vi "纳清pH电极校准.vi"() -> ()   [LabVIEW 2016, in "斯坦道多参数.lvlib"]
uses:
  <vilib>/Utility/miscctls.llb/LVPointTypeDef.ctl
  <vilib>/Utility/miscctls.llb/LVPositionTypeDef.ctl
  <vilib>/Analysis/NI_AALBase.lvlib
panel:
  out "当前探头类别":string
  out "报警信息":string
  out "温度校准参数":sgl format="%#.2f"
  out "通讯状态":string
  out "第二点校准值":dbl
  out "第一点校准值":dbl
  in  "校准停止":bool
  in  "校准启动":bool
  in  "校准模式":enum16{"两点校准", "单点校准"}(ring)
  out "最小值":sgl format="%#.2f"
  out "最大值":sgl format="%#.2f"
  out "波形图表":sgl(graph) caption="历史曲线"
  out "mean":dbl caption="均值" format="%#.2f"
  out "standard deviation":dbl caption="标准差" format="%#.2f"
  out "变异系数":dbl format="%#.6f"
  out "测量值":sgl format="%#.2f"
  out "提示":string
  out "标液2":sgl
  out "标液1":sgl
  out "原始光强数值":sgl caption="信号值" format="%#.6f"
  out "温度":dbl format="%#.2f"
  # "pH电极设定"
  # "℃"
  # "mV"
  # "℃"
  # "请选择校准模式:"
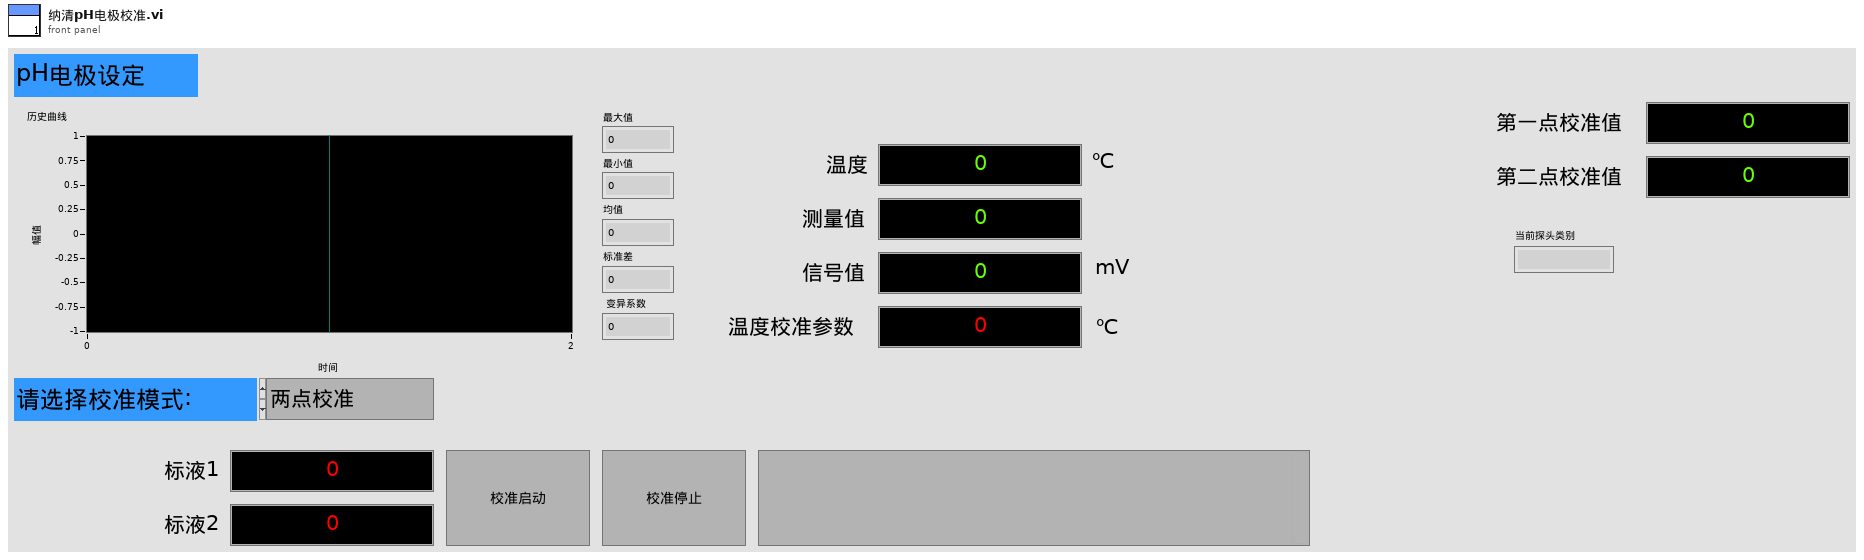
[diagram p1: front panel]
types:
  T1 = typedef "LVPointTypeDef.ctl" = cluster{"Horizontal":i16, "Vertical":i16}
  T2 = typedef "斯坦道多参数.lvlib/校准步骤.ctl" = enum16{"待机", "放置第一点标液", "第一点校准启动", "第一点校准写入", "第一点校准失败", "放置第二点标液", "第二点校准启动", "第二点校准写入", "第二点校准失败", "放置第三点标液", "第三点校准启动", "第三点校准写入", "第三点校准失败", "校准结果写入", "校准结束"}
  T3 = cluster{"报警码":u16, "pH数值":sgl, "0X0003_NC":sgl, "温度数据":sgl, "pH原始信号 mv":sgl, "0X0009_NC":string, "产品名称":string, "序列号":string, "硬件版本":string, "软件版本":string, "通讯地址":u16, "波特率":u16, "设备类型":u16, "0X0026_NC":string, "第一点原始数据":sgl, "第一点校准数据":sgl, "第二点原始数据":sgl, "第二点校准数据":sgl, "探头校准命令":u16, "温度校准参数":sgl, "温度校准命令":u16}
  T4 = typedef "LVPositionTypeDef.ctl" = cluster{"Left":i32, "Top":i32}
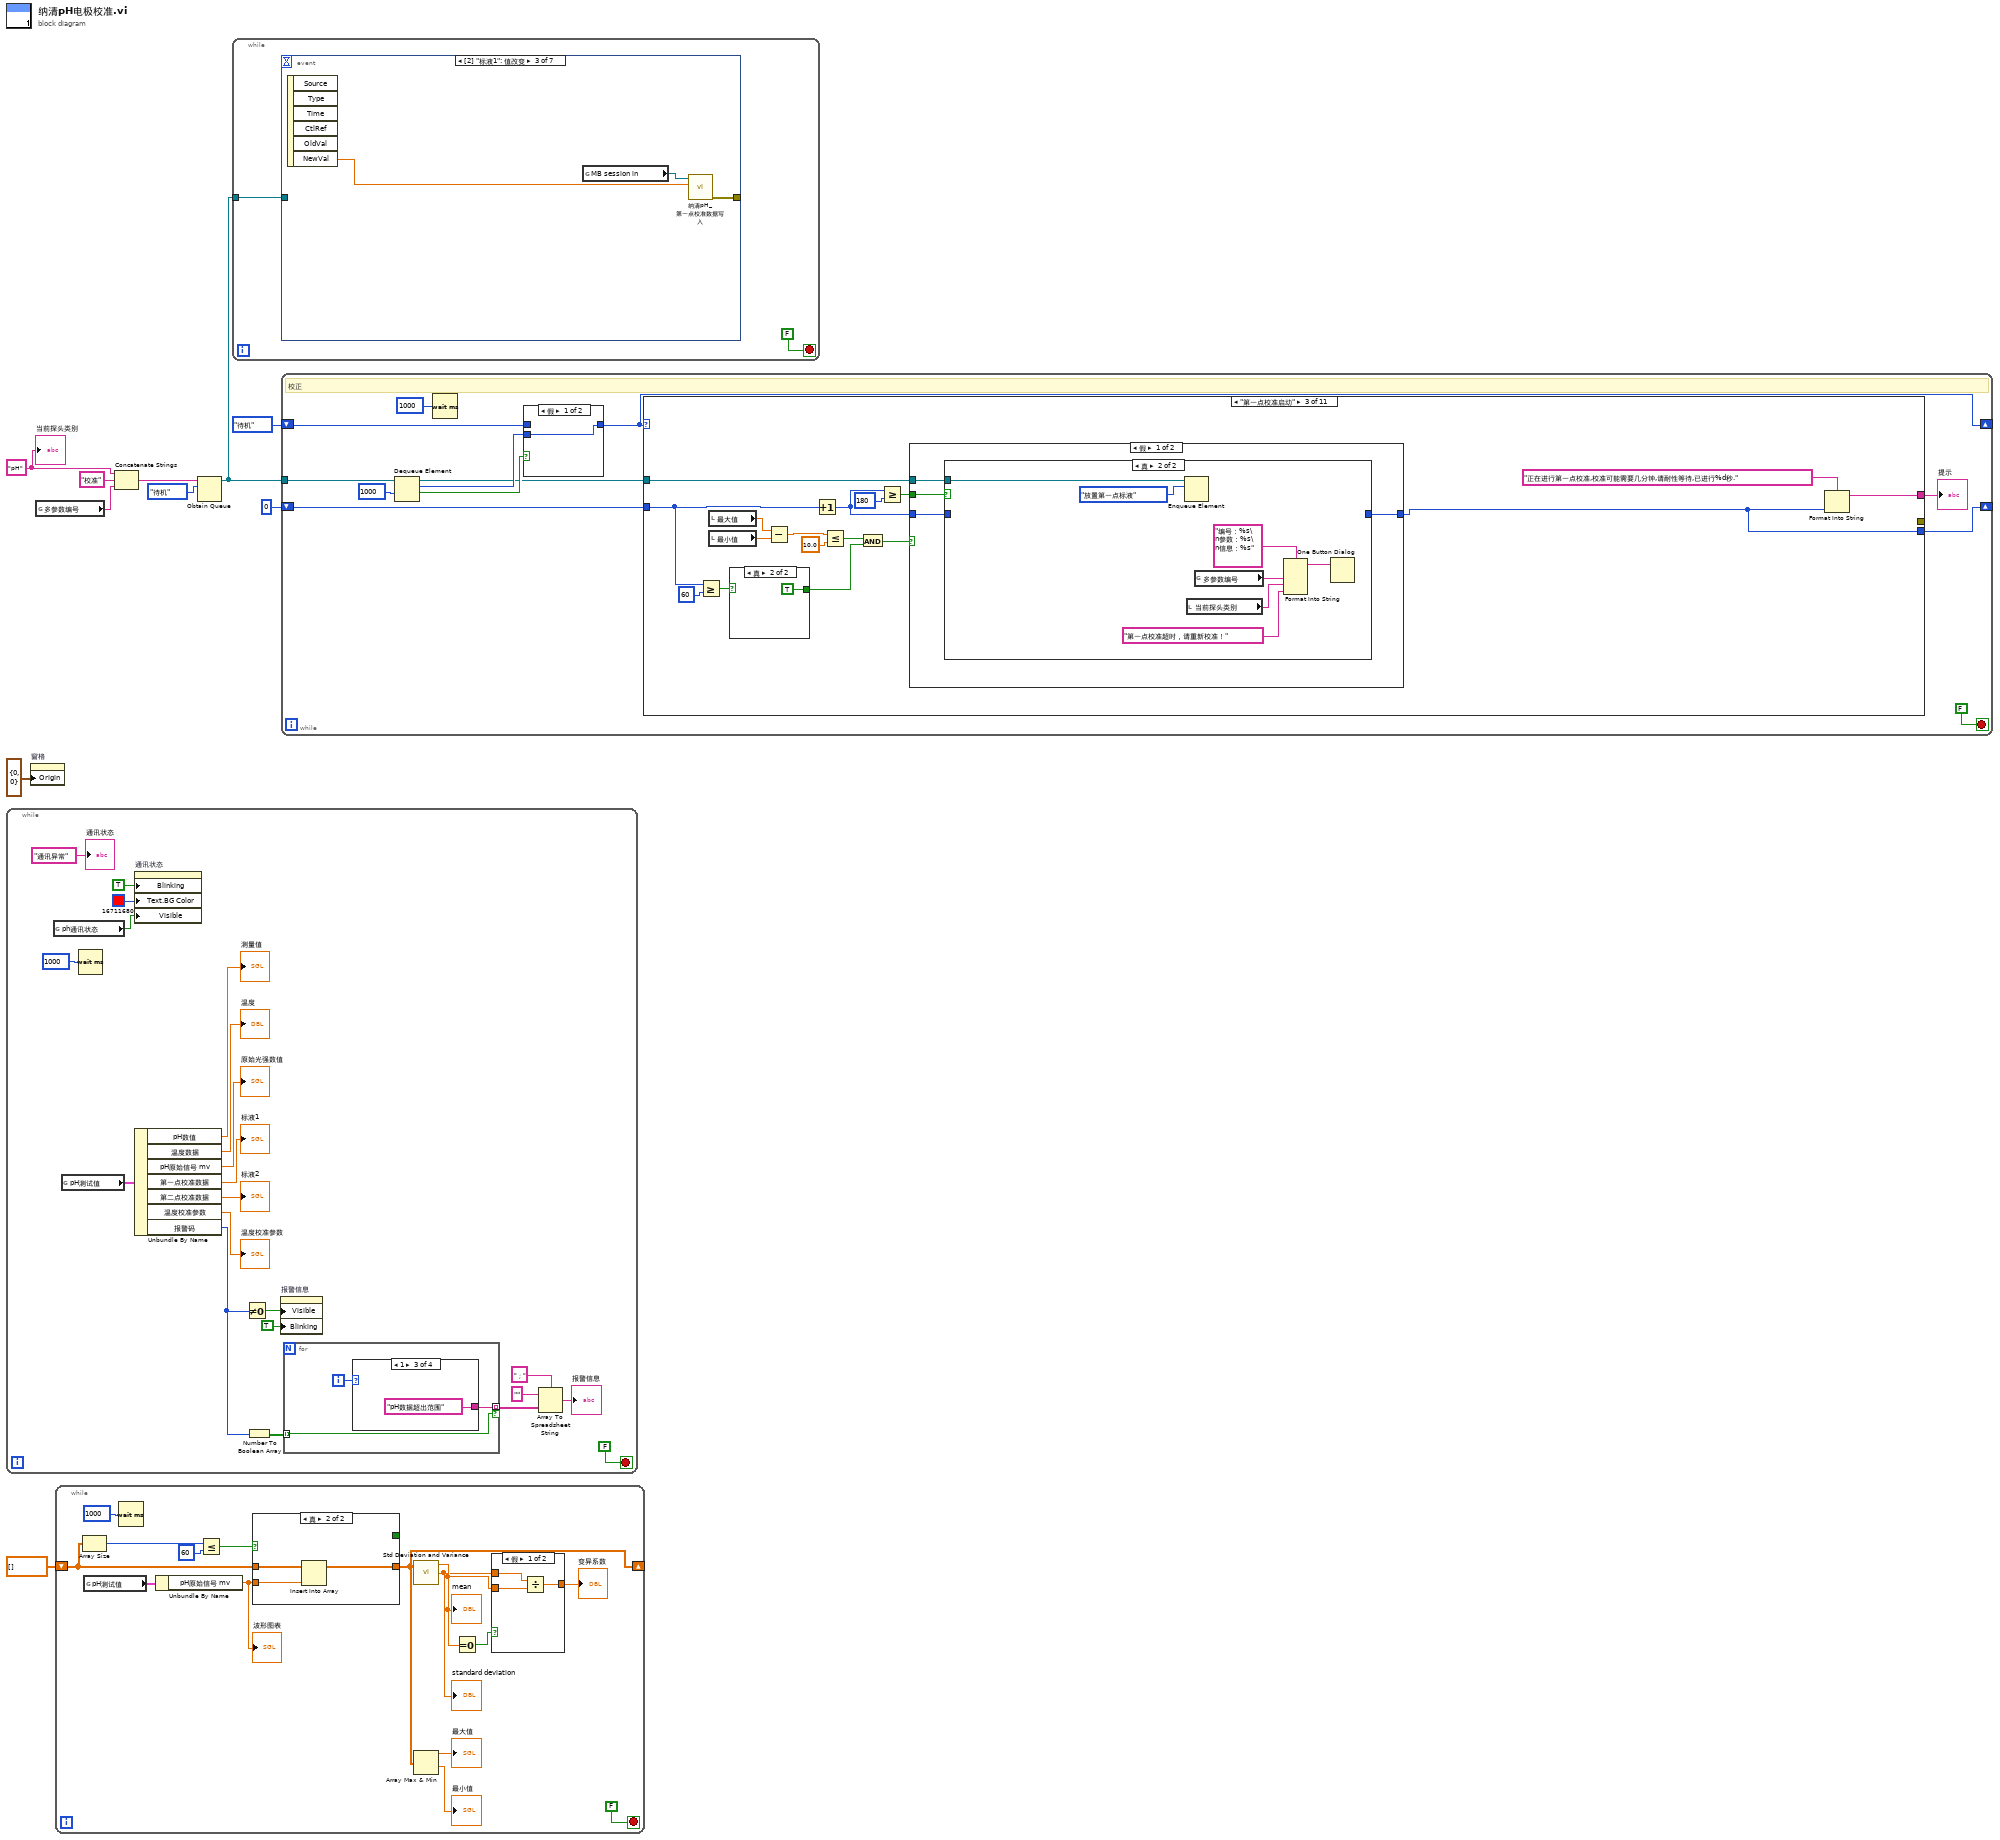
[diagram p0: block diagram]
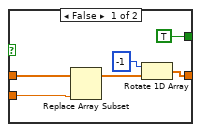
[diagram p3: hidden frame]
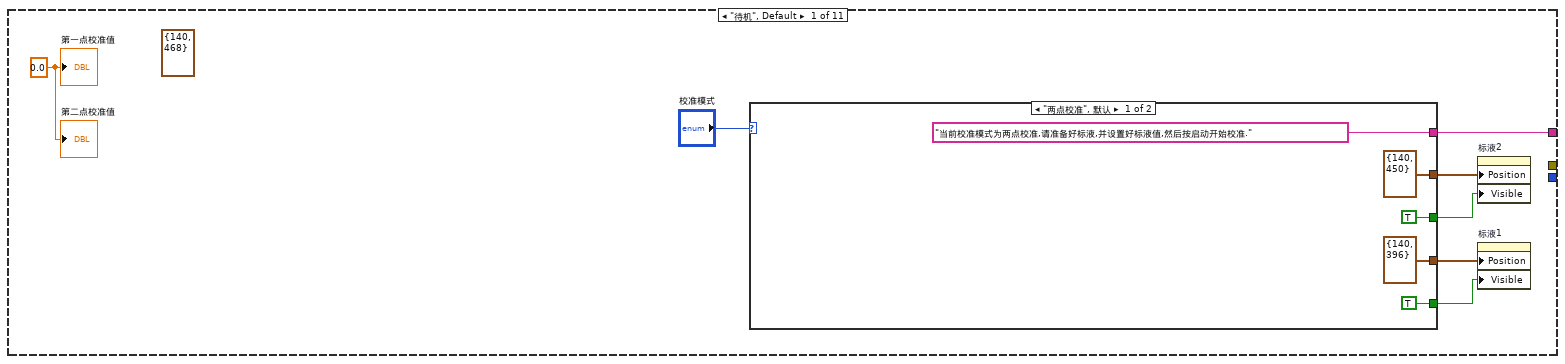
[diagram p5: hidden frame]
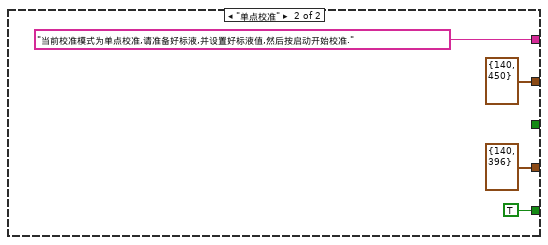
[diagram p6: hidden frame]
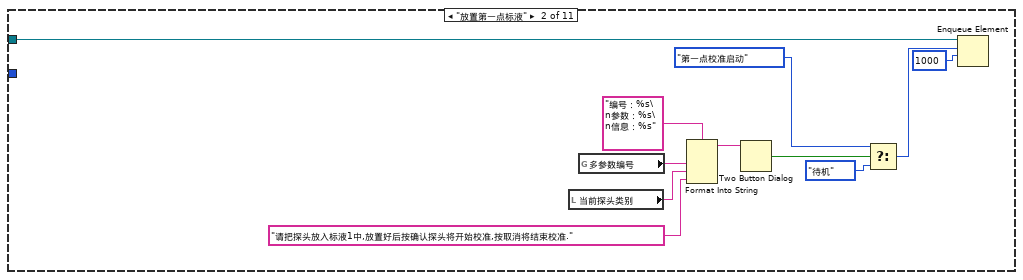
[diagram p7: hidden frame]
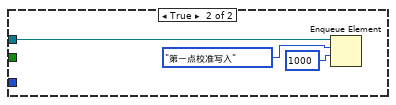
[diagram p9: hidden frame]
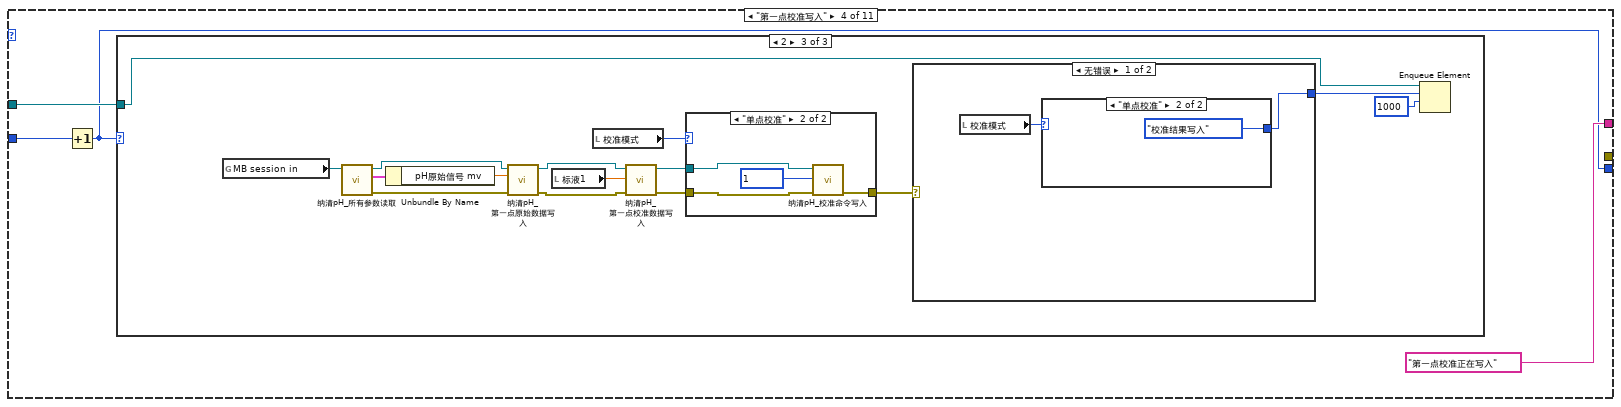
[diagram p11: hidden frame]
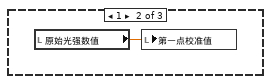
[diagram p13: hidden frame]
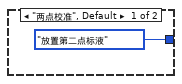
[diagram p15: hidden frame]
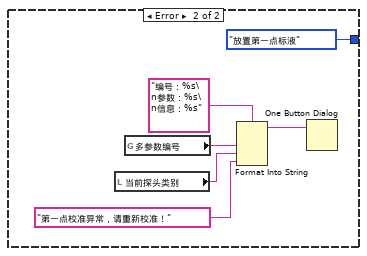
[diagram p16: hidden frame]
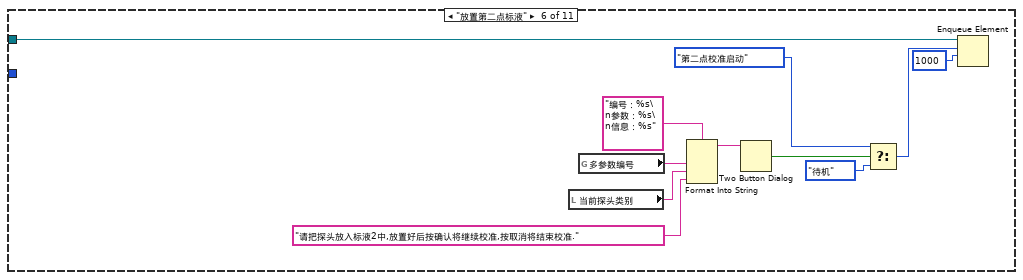
[diagram p18: hidden frame]
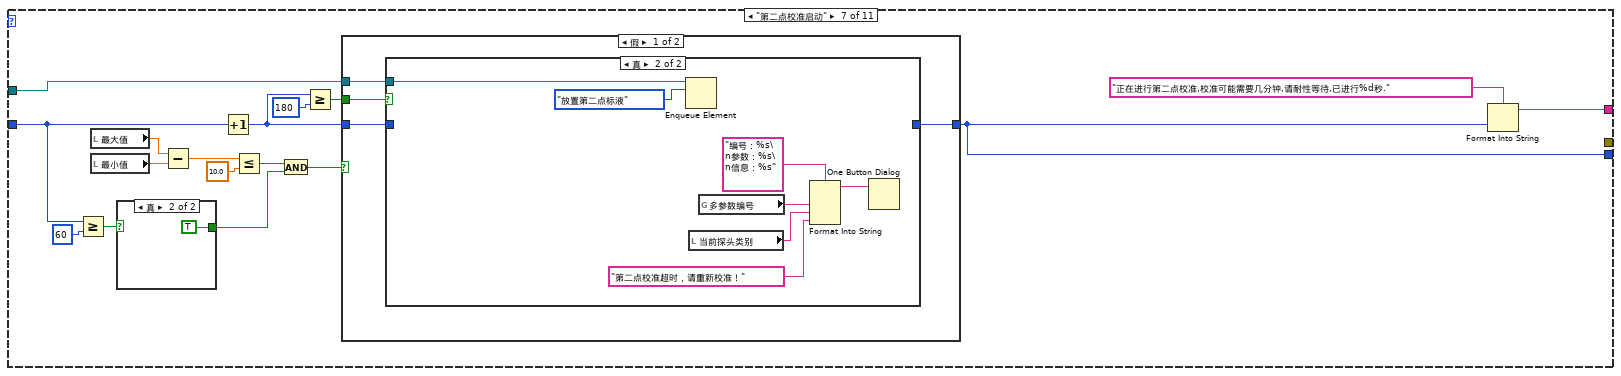
[diagram p19: hidden frame]
diagram:
  w1 = "pH" ("当前探头类别")
  n1 = while {
    stop <- FALSE stop-if-true
    n2 = global read "多参数全局变量.vi" "ph通讯状态"() -> (w20:bool)
    n3 = global read "纳清过程全局变量.vi" "pH测试值"() -> (w29:T3)
    n4 = Wait (ms)(milliseconds to wait=u32 1000 ("等待时间（毫秒）")) -> ()  [unwired: 1 out]
    n5 = property on="通讯状态" class="Str"("Blinking"=TRUE ("闪烁"), "Text.BG Color"=u32 16711680, "Visible"=w20) -> ()  [unwired: 2 in, 2 out]
    n6 = Unbundle By Name(w29) -> ("pH数值"=→"测量值":sgl, "温度数据"=→"温度":sgl, "pH原始信号 mv"=→"原始光强数值":sgl, "第一点校准数据"=→"标液1":sgl, "第二点校准数据"=→"标液2":sgl, "温度校准参数"=→"温度校准参数":sgl, "报警码"=w13:u16)
    n7 = Not Equal To 0?(x=w13) -> (x != 0?=w12:bool)
    n8 = Number To Boolean Array(number=w13) -> (Boolean array=w18:bool[])
    n9 = property on="报警信息" class="Str"("Visible"=w12, "Blinking"=TRUE ("闪烁")) -> ()  [unwired: 2 in, 2 out]
    n10 = for {
      tunnel: w18 -> [w32] mode=indexing
      tunnel: [w33] -> w17 mode=indexing if=w32
      i -> [w34]
      n11 = case shown="1" w34 {
        tunnel: [_ "温度超出范围" "pH数据超出范围" "温度传感器故障"] -> w33
        frame Default {
        }
        frame 0 {
        }
        frame 1 {
        }
        frame 8 {
        }
      }
    }
    n12 = Array To Spreadsheet String(delimiter (Tab)="；" ("分隔符(Tab)"), array=w17, 3:"" ("格式字符串")) -> (spreadsheet string=→"报警信息":string)
    "通讯状态" <- "通讯异常" ("当前串口")
  }
  n13 = property on="窗格" class="Pane"("Origin"=T1 {"Horizontal"=0, "Vertical"=0} ("原点")) -> ()  [unwired: 2 in, 2 out]
  n14 = global read "多参数全局变量.vi" "多参数编号"() -> (w2:string)
  n15 = while {
    shift-right: [w42] -> _
    shift-left: sgl[] [] -> [w48]
    stop <- FALSE stop-if-true
    n16 = Array Size(array=w48) -> (size(s)=w50:i32)
    n17 = global read "纳清过程全局变量.vi" "pH测试值"() -> (w38:T3)
    n18 = Wait (ms)(milliseconds to wait=u32 1000 ("等待时间（毫秒）")) -> ()  [unwired: 1 out]
    n19 = Unbundle By Name(w38) -> ("pH原始信号 mv"=w39:sgl)
    "波形图表" <- w39
    n20 = Less Or Equal?(x=w50, y=60) -> (x <= y?=w49:bool)
    n21 = case shown="真" w49 {
      tunnel: w48 -> [w61 w64]
      tunnel: w39 -> [w59 w63]
      tunnel: [w57 w62] -> w42
      tunnel: [TRUE _] -> _
      frame False {
        n22 = Replace Array Subset(array=w61, new element=w59) -> (w60:sgl[])  [unwired: 1 in]
        n23 = Rotate 1D Array(1:w60, 2:-1 ("n")) -> (0:w57:sgl[])
      }
      frame True {
        n24 = Insert Into Array(array=w64, new element=w63) -> (w62:sgl[])  [unwired: 1 in]
      }
    }
    n25 = call <vilib>:"Std Deviation and Variance.vi"("X"=w42) -> ("mean"=w46:dbl, "standard deviation"=w45:dbl)  [unwired: 1 in, 1 out]
    "mean" <- w46
    "standard deviation" <- w45
    n26 = Array Max & Min(array=w42) -> (max value=→"最大值":sgl, min value=→"最小值":sgl)  [unwired: 2 out]
    n27 = Equal To 0?(x=w46) -> (x = 0?=w47:bool)
    n28 = case shown="假" w47 {
      tunnel: w45 -> [w55 _]
      tunnel: [w54 _] -> w44
      tunnel: w46 -> [w53 _]
      frame False {
        n29 = Divide(x=w55, y=w53) -> (x/y=w54:dbl)
      }
      frame True {
      }
    }
    "变异系数" <- w44
  }
  n30 = Concatenate Strings(w1, "校准" ("名称（未命名）"), w2) -> (w3:string)
  n31 = Obtain Queue(name (unnamed)=w3, element data type=校准步骤."待机" ("枚举")) -> (queue out=w5:refnum<queue>)  [unwired: 3 in, 2 out]
  n32 = while {
    tunnel: w5 -> [w65]
    stop <- FALSE stop-if-true
    n33 = event shown="[2] \"标液1\": 值改变" {
      selector: _ -> [_ _ _ _ _ _ _]
      dyn-events: _ -> [_ _ _ _ _ _ _]
      timeout: _ -> [_ _ _ _ _ _ _]
      tunnel: [_ _ w72 w76 w77 _ _] -> _
      tunnel: w65 -> [_ _ _ _ _ w84 w86]
      event Timeout {
        n34 = event-data() -> ()  [unwired: 1 in, 3 out]
      }
      event "标液1", "标液2", "温度校准参数": Mouse Down {
        n35 = event-data() -> ("CtlRef"=w67:refnum<vi>)  [unwired: 1 in, 7 out]
        n36 = property class="DigNum (严格)"(reference=w67) -> (reference out=w68:refnum<vi>, "Value"=w69:sgl)  [unwired: 1 in, 1 out]
        n37 = call "数字键盘.vi"("OldNumber"=w69) -> ("NewNumber"=w70:dbl)  [unwired: 1 in]
        n38 = property class="DigNum (严格)"(reference=w68, "Val(Sgnl)"=w70) -> ()  [unwired: 1 in, 2 out]
      }
      event "标液1": Value Change {
        n39 = event-data() -> ("NewVal"=w71:sgl)  [unwired: 1 in, 5 out]
        n40 = global read "多参数全局变量.vi" "MB session in"() -> (w73:refnum<class "MB_Master.lvclass">)
        n41 = call "纳清pH_第一点校准数据写入.vi"("数值"=w71, "MB session in"=w73) -> ("error out"=w72:errorcluster)  [unwired: 8 in, 1 out]
      }
      event "标液2": Value Change {
        n42 = event-data() -> ("NewVal"=w75:sgl)  [unwired: 1 in, 5 out]
        n43 = global read "多参数全局变量.vi" "MB session in"() -> (w74:refnum<class "MB_Master.lvclass">)
        n44 = call "纳清pH_第二点校准数据写入.vi"("数值"=w75, "MB session in"=w74) -> ("error out"=w76:errorcluster)  [unwired: 8 in, 1 out]
      }
      event "温度校准参数": Value Change {
        n45 = event-data() -> ("NewVal"=w82:sgl)  [unwired: 1 in, 5 out]
        n46 = global read "多参数全局变量.vi" "MB session in"() -> (w81:refnum<class "MB_Master.lvclass">)
        n47 = call "纳清pH_温度校准参数写入.vi"("数值"=w82, "MB session in"=w81) -> ("error out"=w83:errorcluster, "MB session out"=w80:refnum<class "MB_Master.lvclass">)  [unwired: 8 in]
        n48 = call "纳清pH_温度校准命令写入.vi"("error in (no error)"=w83, "数值"=u16 1 ("starting address"), "MB session in"=w80) -> ("error out"=w78:errorcluster)  [unwired: 7 in, 1 out]
        n49 = call <vilib>:"Simple Error Handler.vi"("error in (no error)"=w78) -> ("error out"=w77:errorcluster)  [unwired: 4 in, 4 out]
      }
      event "校准启动": Value Change {
        n50 = event-data() -> ()  [unwired: 1 in, 6 out]
        n51 = Enqueue Element(queue=w84, element=校准步骤."放置第一点标液" ("元素")) -> ()  [unwired: 2 in, 3 out]
      }
      event "校准停止": Value Change {
        n52 = event-data() -> ()  [unwired: 1 in, 6 out]
        n53 = Flush Queue(queue=w86) -> (queue out=w87:refnum<queue>)  [unwired: 1 in, 2 out]
        n54 = Enqueue Element(queue=w87, element=校准步骤."待机" ("元素"), timeout in ms (-1)=1000 ("超时毫秒(-1)")) -> ()  [unwired: 1 in, 3 out]
      }
    }
  }
  n55 = while "While循环" {
    shift-right: [w91] -> _
    shift-left: 校准步骤."待机" ("枚举") -> [w93]
    shift-right: [w90] -> _
    shift-left: 0 -> [w99]
    tunnel: w5 -> [w94]
    stop <- FALSE stop-if-true
    # "校正"
    n56 = Dequeue Element(queue=w94, timeout in ms (-1)=1000 ("超时毫秒(-1)")) -> (queue out=w92:refnum<queue>, element=w95:T2, timed out?=w96:bool)  [unwired: 1 in, 1 out]
    n57 = Wait (ms)(milliseconds to wait=u32 1000 ("等待时间（毫秒）")) -> ()  [unwired: 1 out]
    n58 = case shown="假" w96 {
      tunnel: w95 -> [w102 _]
      tunnel: [w102 w103] -> w91
      tunnel: w93 -> [_ w103]
      frame False {
      }
      frame True {
      }
    }
    n59 = case shown="\"第一点校准启动\"" w91 {
      tunnel: [w109 _ w132 "第一点校准正在写入" ("提示") _ _ w212 "第二点校准正在写入" ("提示") "第二点校准失败" ("提示") w281 w299] -> w98
      tunnel: w99 -> [_ _ w133 w166 _ _ w213 w245 _ _ _]
      tunnel: [_ _ w131 w164 _ _ w211 w243 _ _ _] -> w90
      tunnel: w92 -> [_ w126 w134 w165 _ w204 w214 w244 _ w287 _]
      tunnel: [_ _ _ _ _ _ _ _ _ w285 _] -> _
      frame "待机", Default {
        (unwired) T4 {"Left"=140, "Top"=468} ("位置 3")
        w104 = 0.0 ("第一点校准值")
        n60 = case shown="\"两点校准\", 默认" "校准模式" {
          tunnel: ["当前校准模式为两点校准,请准备好标液,并设置好标液值,然后按启动开始校准." ("提示") "当前校准模式为单点校准,请准备好标液,并设置好标液值,然后按启动开始校准." ("提示")] -> w109
          tunnel: [TRUE ("可见") _] -> w106
          tunnel: [T4 {"Left"=140, "Top"=396} ("位置") T4 {"Left"=140, "Top"=396} ("位置")] -> w108
          tunnel: [T4 {"Left"=140, "Top"=450} ("位置 2") T4 {"Left"=140, "Top"=450} ("位置 2")] -> w107
          tunnel: [TRUE ("可见") TRUE ("可见")] -> w105
          frame "两点校准", Default {
          }
          frame "单点校准" {
          }
        }
        n61 = property on="标液2" class="DigNum (严格)"("Position"=w107, "Visible"=w106) -> ()  [unwired: 2 in, 2 out]
        n62 = property on="标液1" class="DigNum (严格)"("Position"=w108, "Visible"=w105) -> ()  [unwired: 2 in, 2 out]
        "第一点校准值" <- w104
        "第二点校准值" <- w104
      }
      frame "放置第一点标液" {
        n63 = local read "当前探头类别"() -> (w120:string)
        n64 = global read "多参数全局变量.vi" "多参数编号"() -> (w124:string)
        n65 = Format Into String(format string="编号：%s\n参数：%s\n信息：%s" ("格式字符串"), w124, w120, "请把探头放入标液1中,放置好后按确认探头将开始校准,按取消将结束校准." ("消息")) -> (resulting string=w123:string)  [unwired: 2 in, 1 out]
        n66 = Two Button Dialog(message=w123) -> (T button?=w121:bool)  [unwired: 2 in]
        n67 = Select(t=校准步骤."第一点校准启动" ("元素"), s=w121, f=校准步骤."待机" ("元素")) -> (s? t:f=w127:T2)
        n68 = Enqueue Element(queue=w126, element=w127, timeout in ms (-1)=1000 ("超时毫秒(-1)")) -> ()  [unwired: 1 in, 3 out]
      }
      frame "第一点校准启动" {
        n69 = Greater Or Equal?(x=w133, y=60) -> (x >= y?=w140:bool)
        n70 = local read "最大值"() -> (w143:sgl)
        n71 = local read "最小值"() -> (w142:sgl)
        n72 = case shown="真" w140 {
          tunnel: [_ TRUE] -> w141
          frame False {
          }
          frame True {
          }
        }
        n73 = Subtract(x=w143, y=w142) -> (x-y=w144:sgl)
        n74 = Increment(x=w133) -> (x+1=w147:i32)
        n75 = Less Or Equal?(x=w144, y=10.0) -> (x <= y?=w137:bool)
        n76 = And(x=w137, y=w141) -> (x .and. y?=w145:bool)
        n77 = Greater Or Equal?(x=w147, y=180) -> (x >= y?=w146:bool)
        n78 = case shown="假" w145 {
          tunnel: w134 -> [w150 w162]
          tunnel: w146 -> [w151 _]
          tunnel: w147 -> [w149 _]
          tunnel: [w148 _] -> w131
          frame False {
            n79 = case shown="真" w151 {
              tunnel: w150 -> [_ w159]
              tunnel: w149 -> [w152 _]
              tunnel: [w152 _] -> w148
              frame False {
              }
              frame True {
                n80 = Enqueue Element(queue=w159, element=校准步骤."放置第一点标液" ("元素")) -> ()  [unwired: 2 in, 3 out]
                n81 = local read "当前探头类别"() -> (w153:string)
                n82 = global read "多参数全局变量.vi" "多参数编号"() -> (w156:string)
                n83 = Format Into String(format string="编号：%s\n参数：%s\n信息：%s" ("格式字符串"), w156, w153, "第一点校准超时，请重新校准！" ("error source (\" \")")) -> (resulting string=w154:string)  [unwired: 2 in, 1 out]
                n84 = One Button Dialog(message=w154) -> ()  [unwired: 1 in, 1 out]
              }
            }
          }
          frame True {
            n85 = Enqueue Element(queue=w162, element=校准步骤."第一点校准写入" ("元素"), timeout in ms (-1)=1000 ("超时毫秒(-1)")) -> ()  [unwired: 1 in, 3 out]
          }
        }
        n86 = Format Into String(format string="正在进行第一点校准,校准可能需要几分钟,请耐性等待,已进行%d秒." ("格式字符串"), w131) -> (resulting string=w132:string)  [unwired: 2 in, 1 out]
      }
      frame "第一点校准写入" {
        n87 = Increment(x=w166) -> (x+1=w164:i32)
        n88 = case shown="2" w164 {
          tunnel: w165 -> [_ _ w183]
          frame 0, Default {
          }
          frame 1 {
            n89 = local read "原始光强数值"() -> (w168:sgl)
            n90 = local write "第一点校准值"(w168) -> ()
          }
          frame 2 {
            n91 = global read "多参数全局变量.vi" "MB session in"() -> (w179:refnum<class "MB_Master.lvclass">)
            n92 = call "纳清pH_所有参数读取.vi"("MB session in"=w179) -> ("error out"=w181:errorcluster, "输出值"=w178:T3, "MB session out"=w180:refnum<class "MB_Master.lvclass">)  [unwired: 8 in]
            n93 = Unbundle By Name(w178) -> ("pH原始信号 mv"=w177:sgl)
            n94 = call "纳清pH_第一点原始数据写入.vi"("error in (no error)"=w181, "数值"=w177, "MB session in"=w180) -> ("error out"=w176:errorcluster, "MB session out"=w175:refnum<class "MB_Master.lvclass">)  [unwired: 7 in]
            n95 = local read "标液1"() -> (w172:sgl)
            n96 = local read "校准模式"() -> (w169:enum16{"两点校准", "单点校准"})
            n97 = call "纳清pH_第一点校准数据写入.vi"("error in (no error)"=w176, "数值"=w172, "MB session in"=w175) -> ("error out"=w174:errorcluster, "MB session out"=w173:refnum<class "MB_Master.lvclass">)  [unwired: 7 in]
            n98 = case shown="\"单点校准\"" w169 {
              tunnel: w174 -> [w184 w188]
              tunnel: w173 -> [_ w187]
              tunnel: [w184 w185] -> w171
              frame "两点校准", Default {
              }
              frame "单点校准" {
                n99 = call "纳清pH_校准命令写入.vi"("error in (no error)"=w188, "数值"=u16 1 ("starting address"), "MB session in"=w187) -> ("error out"=w185:errorcluster)  [unwired: 7 in, 1 out]
              }
            }
            n100 = case shown="无错误" w171 {
              tunnel: [w189 校准步骤."放置第一点标液" ("元素")] -> w170
              frame No Error {
                n101 = local read "校准模式"() -> (w190:enum16{"两点校准", "单点校准"})
                n102 = case shown="\"单点校准\"" w190 {
                  tunnel: [校准步骤."放置第二点标液" ("元素") 校准步骤."校准结果写入" ("元素")] -> w189
                  frame "两点校准", Default {
                  }
                  frame "单点校准" {
                  }
                }
              }
              frame Error {
                n103 = local read "当前探头类别"() -> (w193:string)
                n104 = global read "多参数全局变量.vi" "多参数编号"() -> (w197:string)
                n105 = Format Into String(format string="编号：%s\n参数：%s\n信息：%s" ("格式字符串"), w197, w193, "第一点校准异常，请重新校准！" ("error source (\" \")")) -> (resulting string=w195:string)  [unwired: 2 in, 1 out]
                n106 = One Button Dialog(message=w195) -> ()  [unwired: 1 in, 1 out]
              }
            }
            n107 = Enqueue Element(queue=w183, element=w170, timeout in ms (-1)=1000 ("超时毫秒(-1)")) -> ()  [unwired: 1 in, 3 out]
          }
        }
      }
      frame "第一点校准失败" {
      }
      frame "放置第二点标液" {
        n108 = local read "当前探头类别"() -> (w199:string)
        n109 = global read "多参数全局变量.vi" "多参数编号"() -> (w202:string)
        n110 = Format Into String(format string="编号：%s\n参数：%s\n信息：%s" ("格式字符串"), w202, w199, "请把探头放入标液2中,放置好后按确认将继续校准,按取消将结束校准." ("消息")) -> (resulting string=w201:string)  [unwired: 2 in, 1 out]
        n111 = Two Button Dialog(message=w201) -> (T button?=w208:bool)  [unwired: 2 in]
        n112 = Select(t=校准步骤."第二点校准启动" ("元素"), s=w208, f=校准步骤."待机" ("元素")) -> (s? t:f=w205:T2)
        n113 = Enqueue Element(queue=w204, element=w205, timeout in ms (-1)=1000 ("超时毫秒(-1)")) -> ()  [unwired: 1 in, 3 out]
      }
      frame "第二点校准启动" {
        n114 = Greater Or Equal?(x=w213, y=60) -> (x >= y?=w219:bool)
        n115 = local read "最大值"() -> (w222:sgl)
        n116 = local read "最小值"() -> (w221:sgl)
        n117 = case shown="真" w219 {
          tunnel: [_ TRUE] -> w220
          frame False {
          }
          frame True {
          }
        }
        n118 = Subtract(x=w222, y=w221) -> (x-y=w223:sgl)
        n119 = Increment(x=w213) -> (x+1=w226:i32)
        n120 = Less Or Equal?(x=w223, y=10.0) -> (x <= y?=w216:bool)
        n121 = And(x=w216, y=w220) -> (x .and. y?=w224:bool)
        n122 = Greater Or Equal?(x=w226, y=180) -> (x >= y?=w225:bool)
        n123 = case shown="假" w224 {
          tunnel: w214 -> [w229 w241]
          tunnel: w225 -> [w230 _]
          tunnel: w226 -> [w228 _]
          tunnel: [w227 _] -> w211
          frame False {
            n124 = case shown="真" w230 {
              tunnel: w229 -> [_ w238]
              tunnel: w228 -> [w231 _]
              tunnel: [w231 _] -> w227
              frame False {
              }
              frame True {
                n125 = Enqueue Element(queue=w238, element=校准步骤."放置第二点标液" ("元素")) -> ()  [unwired: 2 in, 3 out]
                n126 = local read "当前探头类别"() -> (w232:string)
                n127 = global read "多参数全局变量.vi" "多参数编号"() -> (w235:string)
                n128 = Format Into String(format string="编号：%s\n参数：%s\n信息：%s" ("格式字符串"), w235, w232, "第二点校准超时，请重新校准！" ("消息")) -> (resulting string=w234:string)  [unwired: 2 in, 1 out]
                n129 = One Button Dialog(message=w234) -> ()  [unwired: 1 in, 1 out]
              }
            }
          }
          frame True {
            n130 = Enqueue Element(queue=w241, element=校准步骤."第二点校准写入" ("元素"), timeout in ms (-1)=1000 ("超时毫秒(-1)")) -> ()  [unwired: 1 in, 3 out]
          }
        }
        n131 = Format Into String(format string="正在进行第二点校准,校准可能需要几分钟,请耐性等待,已进行%d秒." ("格式字符串"), w211) -> (resulting string=w212:string)  [unwired: 2 in, 1 out]
      }
      frame "第二点校准写入" {
        n132 = Increment(x=w245) -> (x+1=w243:i32)
        n133 = case shown="2" w243 {
          tunnel: w244 -> [_ _ w262]
          frame 0, Default {
          }
          frame 1 {
            n134 = local read "原始光强数值"() -> (w247:sgl)
            n135 = local write "第二点校准值"(w247) -> ()
          }
          frame 2 {
            n136 = global read "多参数全局变量.vi" "MB session in"() -> (w258:refnum<class "MB_Master.lvclass">)
            n137 = call "纳清pH_所有参数读取.vi"("MB session in"=w258) -> ("error out"=w260:errorcluster, "输出值"=w257:T3, "MB session out"=w259:refnum<class "MB_Master.lvclass">)  [unwired: 8 in]
            n138 = Unbundle By Name(w257) -> ("pH原始信号 mv"=w256:sgl)
            n139 = call "纳清pH_第二点原始数据写入.vi"("error in (no error)"=w260, "数值"=w256, "MB session in"=w259) -> ("error out"=w255:errorcluster, "MB session out"=w254:refnum<class "MB_Master.lvclass">)  [unwired: 7 in]
            n140 = local read "标液2"() -> (w251:sgl)
            n141 = local read "校准模式"() -> (w248:enum16{"两点校准", "单点校准"})
            n142 = call "纳清pH_第二点校准数据写入.vi"("error in (no error)"=w255, "数值"=w251, "MB session in"=w254) -> ("error out"=w253:errorcluster, "MB session out"=w252:refnum<class "MB_Master.lvclass">)  [unwired: 7 in]
            n143 = case shown="\"两点校准\"" w248 {
              tunnel: w253 -> [w266 w267]
              tunnel: w252 -> [w265 _]
              tunnel: [w263 w267] -> w250
              frame "两点校准" {
                n144 = call "纳清pH_校准命令写入.vi"("error in (no error)"=w266, "数值"=u16 2 ("starting address"), "MB session in"=w265) -> ("error out"=w263:errorcluster)  [unwired: 7 in, 1 out]
              }
              frame "单点校准", Default {
              }
            }
            n145 = case shown="错误" w250 {
              tunnel: [w268 校准步骤."放置第二点标液" ("元素")] -> w249
              frame No Error {
                n146 = local read "校准模式"() -> (w269:enum16{"两点校准", "单点校准"})
                n147 = case shown="\"单点校准\"" w269 {
                  tunnel: [校准步骤."校准结果写入" ("元素") 校准步骤."校准结果写入" ("元素")] -> w268
                  frame "两点校准", Default {
                  }
                  frame "单点校准" {
                  }
                }
              }
              frame Error {
                n148 = local read "当前探头类别"() -> (w272:string)
                n149 = global read "多参数全局变量.vi" "多参数编号"() -> (w276:string)
                n150 = Format Into String(format string="编号：%s\n参数：%s\n信息：%s" ("格式字符串"), w276, w272, "第二点校准异常，请重新校准！" ("error source (\" \")")) -> (resulting string=w274:string)  [unwired: 2 in, 1 out]
                n151 = One Button Dialog(message=w274) -> ()  [unwired: 1 in, 1 out]
              }
            }
            n152 = Enqueue Element(queue=w262, element=w249, timeout in ms (-1)=1000 ("超时毫秒(-1)")) -> ()  [unwired: 1 in, 3 out]
          }
        }
      }
      frame "第二点校准失败" {
      }
      frame "校准结果写入" {
        n153 = Enqueue Element(queue=w287, element=校准步骤."校准结束" ("元素")) -> ()  [unwired: 2 in, 3 out]
        n154 = local read "校准模式"() -> (w286:enum16{"两点校准", "单点校准"})
        n155 = case shown="\"单点校准\"" w286 {
          tunnel: [w291 w298] -> w282
          frame "两点校准", Default {
            n156 = local read "第一点校准值"() -> (w294:dbl)
            n157 = local read "第二点校准值"() -> (w290:dbl)
            n158 = local read "标液1"() -> (w292:sgl)
            n159 = local read "标液2"() -> (w289:sgl)
            n160 = Format Into String(format string="校准结果：第一点校准值=%f，第一点标准值=%f,第二点校准值=%f，第二点标准值=%f." ("提示"), w294, w292, w290, w289) -> (resulting string=w291:string)  [unwired: 2 in, 1 out]
          }
          frame "单点校准" {
            n161 = local read "第一点校准值"() -> (w297:dbl)
            n162 = local read "标液1"() -> (w295:sgl)
            n163 = Format Into String(format string="校准结果：校准值=%f，标准值=%f。" ("提示"), w297, w295) -> (resulting string=w298:string)  [unwired: 2 in, 1 out]
          }
        }
        n164 = local read "当前探头类别"() -> (w279:string)
        n165 = global read "多参数全局变量.vi" "多参数编号"() -> (w283:string)
        n166 = Format Into String(format string="编号：%s\n参数：%s\n信息：%s" ("格式字符串"), w283, w279, w282) -> (resulting string=w281:string)  [unwired: 2 in, 1 out]
        n167 = One Button Dialog(message=w281) -> ()  [unwired: 1 in, 1 out]
        n168 = call "操作日志.vi"("table"="校准记录", "日志信息"=w281) -> ("error out"=w285:errorcluster)  [unwired: 9 in]
      }
      frame "校准结束" {
        n169 = local read "提示"() -> (w299:string)
      }
    }
    "提示" <- w98
  }
  "当前探头类别" <- w1
